vi "Close Instrument.vi"(7 "Go Local (\"@LOC\")":bool=TRUE, 8 "error in (no error)":errorcluster, 11 "VNA-PNA in":refnum<class "VNA-PNA.lvclass">) -> (0 "error out":errorcluster, 3 "VNA-PNA out":refnum<class "VNA-PNA.lvclass">)   [LabVIEW 2020, in "VNA-PNA.lvclass"]
uses:
  VNA-PNA.lvclass
  C:/Sandbox/Git_Sandbox/WiSpry Test Framework source code (LV20)/WiSpry Test Framework/Instruments/Instrument.lvclass
  Instrument.lvclass/Instrument.ctl
  Instrument.lvclass
  <instrlib>/Agilent PNA Series/Agilent PNA Series.lvlib
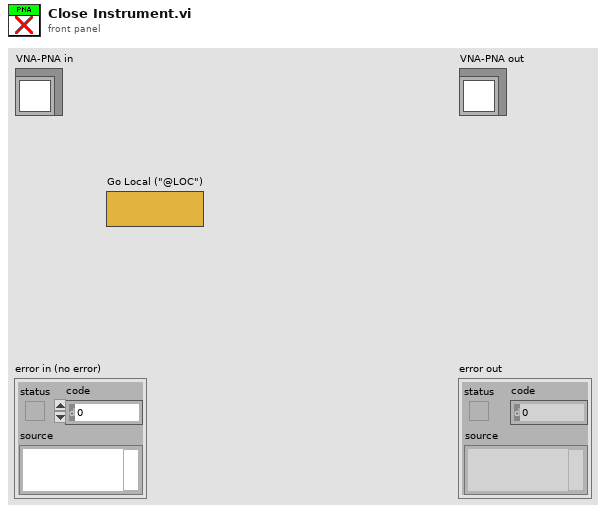
[diagram p1: front panel]
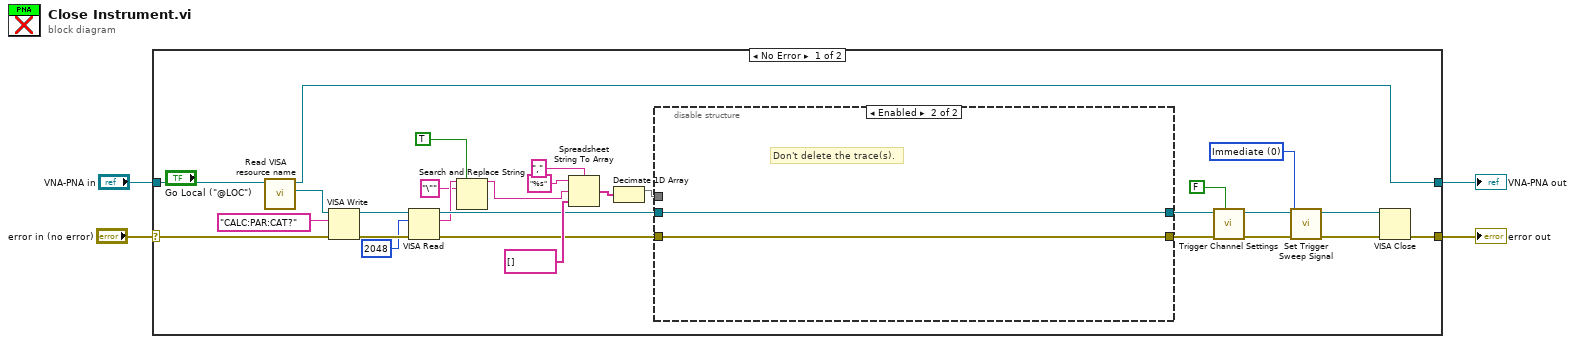
[diagram p0: block diagram]
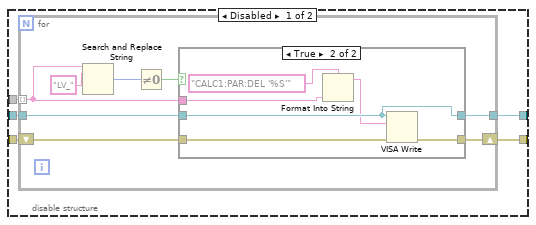
[diagram p2: hidden frame]
diagram:
  n1 = case shown="No Error" "error in (no error)" {
    selector: "error in (no error)" -> [w31 w56]
    tunnel: "VNA-PNA in" -> [w32 w57]
    tunnel: [w13 w56] -> w1
    tunnel: [w14 w57] -> w2
    frame No Error {
      w6 = u16 0 items=["Immediate", "External", "Manual"] ("Source (0: Immediate)")
      n2 = call "Read VISA resource name.vi"("Instrument in"=w32) -> ("VISA resource name"=w30:refnum<visa-resource-name>, "Instrument out"=w14:refnum<class "VNA-PNA.lvclass">)  [unwired: 9 in]
      n3 = VISA Write(VISA resource name=w30, write buffer="CALC:PAR:CAT?", error in (no error)=w31) -> (VISA resource name out=w27:refnum<visa-resource-name>, error out=w28:errorcluster)  [unwired: 1 out]
      n4 = VISA Read(VISA resource name=w27, byte count=u32 2048, error in (no error)=w28) -> (VISA resource name out=w21:refnum<visa-resource-name>, read buffer=w19:string, error out=w20:errorcluster)  [unwired: 1 out]
      n5 = Search and Replace String(replace all?=TRUE ("replace all? (F)"), input string=w19, search string="\"") -> (result string=w17:string)  [unwired: 5 in, 3 out]
      n6 = Spreadsheet String To Array(delimiter (Tab)=",", format string="%s", spreadsheet string=w17, array type (2D Dbl)=string[] []) -> (array=w22:string[])
      n7 = Decimate 1D Array(w22) -> (w15:string[])  [unwired: 1 out]
      n8 = disable-structure shown="Enabled" {
        disable-tunnel: w21 -> [w37 w55]
        disable-tunnel: w20 -> [w36 w54]
        disable-tunnel: w15 -> [w35 _]
        disable-tunnel: [w34 w54] -> w8
        disable-tunnel: [w33 w55] -> w7
        frame Disabled {
          n9 = for {
            tunnel: w37 -> [w42]
            shift-right: [w39] -> w34
            shift-left: w36 -> [w41]
            tunnel: w35 -> [w40] mode=indexing
            tunnel: [w38] -> w33
            n10 = Search and Replace String(input string=w40, search string="LV_") -> (number of replacements=w44:i32)  [unwired: 6 in, 3 out]
            n11 = Not Equal To 0?(x=w44) -> (x != 0?=w43:bool)
            n12 = case shown="True" w43 {
              tunnel: w42 -> [w46 w52]
              tunnel: w41 -> [w47 w51]
              tunnel: w40 -> [_ w53]
              tunnel: [w47 w50] -> w39
              tunnel: [w46 w52] -> w38
              frame False {
              }
              frame True {
                n13 = Format Into String(format string="CALC1:PAR:DEL '%S'" ("string"), w53) -> (resulting string=w48:string)  [unwired: 2 in, 1 out]
                n14 = VISA Write(VISA resource name=w52, write buffer=w48, error in (no error)=w51) -> (error out=w50:errorcluster)  [unwired: 2 out]
              }
            }
          }
        }
        frame Enabled {
          # "Don't delete the trace(s)."
        }
      }
      n15 = call <instrlib>:"Trigger Channel Settings.vi"("Trigger Point (T: On)"=FALSE, "Error In (no error)"=w8, "VISA session"=w7) -> ("Error Out"=w11:errorcluster, "dup VISA session"=w12:refnum<visa-resource-name>)  [unwired: 7 in]
      n16 = call <instrlib>:"Set Trigger Sweep Signal.vi"("Error In (no error)"=w11, "Source (0: Immediate)"=w6, "VISA session"=w12) -> ("Error Out"=w9:errorcluster, "dup VISA session"=w10:refnum<visa-resource-name>)  [unwired: 7 in]
      n17 = VISA Close(VISA resource name=w10, error in (no error)=w9) -> (error out=w13:errorcluster)
    }
    frame Error {
    }
  }
  "error out" <- w1
  "VNA-PNA out" <- w2
